vi "wd_replaceAll (STR).vi"(7 "data":string[](array[string]), 8 "error in (no error)":errorcluster, 9 "channel index":i32, 10 "data type":T7, 11 "meta in":T1={"TargetFile"=path "", "StreamMode"=enum."File", "Append?"=FALSE, "ChunkSize"=0, "TimeColumnMode"=enum."Empty", "TimestampFormat"="", "AbsoluteTime?"=FALSE, "FileAttribute "={"Creator"="", "Title"="", "SheetName"=""}, "Column"=[], "FileRef"=refnum, "MemoryRef"=[], "RecordInfo"=[], " ChannelPreviousInfo"=[], "ChannelFirstRecord"=[], "PredefinedFormattedValueLength"=20, "DiskTemplate"={"XMLRef"=[refnum, refnum, refnum, refnum, refnum, refnum], "ZipPath"=path "", "MetaFile"={"Ref"=refnum, "NextRow"=0, "NextPosition"=0, "Block"=[]}, "TempFolder"=path ""}}) -> (0 "error out":errorcluster, 3 "meta out":T1={"TargetFile"=path "", "StreamMode"=enum."File", "Append?"=FALSE, "ChunkSize"=0, "TimeColumnMode"=enum."Empty", "TimestampFormat"="", "AbsoluteTime?"=FALSE, "FileAttribute "={"Creator"="", "Title"="", "SheetName"=""}, "Column"=[], "FileRef"=refnum, "MemoryRef"=[], "RecordInfo"=[], " ChannelPreviousInfo"=[], "ChannelFirstRecord"=[], "PredefinedFormattedValueLength"=20, "DiskTemplate"={"XMLRef"=[refnum, refnum, refnum, refnum, refnum, refnum], "ZipPath"=path "", "MetaFile"={"Ref"=refnum, "NextRow"=0, "NextPosition"=0, "Block"=[]}, "TempFolder"=path ""}})   [LabVIEW 2017, in "NI_ExcelFile.lvlib"]
uses:
  <vilib>/express/express shared/NI_ExcelFile/NI_ExcelFile.lvlib
  <vilib>/express/express shared/NI_ExcelFile/Ctrls/DataType.ctl
  <vilib>/express/express shared/NI_ExcelFile/Ctrls/MainData.ctl
  <vilib>/express/express shared/NI_ExcelFile/Ctrls/StreamMode.ctl
  <vilib>/express/express shared/NI_ExcelFile/Ctrls/TimeColumnMode.ctl
  <vilib>/express/express shared/NI_ExcelFile/Ctrls/FileAttribute.ctl
  <vilib>/express/express shared/NI_ExcelFile/Ctrls/Columns.ctl
  <vilib>/express/express shared/NI_ExcelFile/Ctrls/ColumnInfo.ctl
  <vilib>/express/express shared/NI_ExcelFile/Ctrls/wd_recordInfo.ctl
  <vilib>/express/express shared/NI_ExcelFile/Ctrls/disk_TemplateFile.ctl
  <vilib>/express/express shared/NI_ExcelFile/Ctrls/meta_file.ctl
  <vilib>/express/express shared/NI_ExcelFile/Ctrls/meta_Block.ctl
  <vilib>/express/express shared/NI_ExcelFile/Ctrls/meta_BlockType.ctl
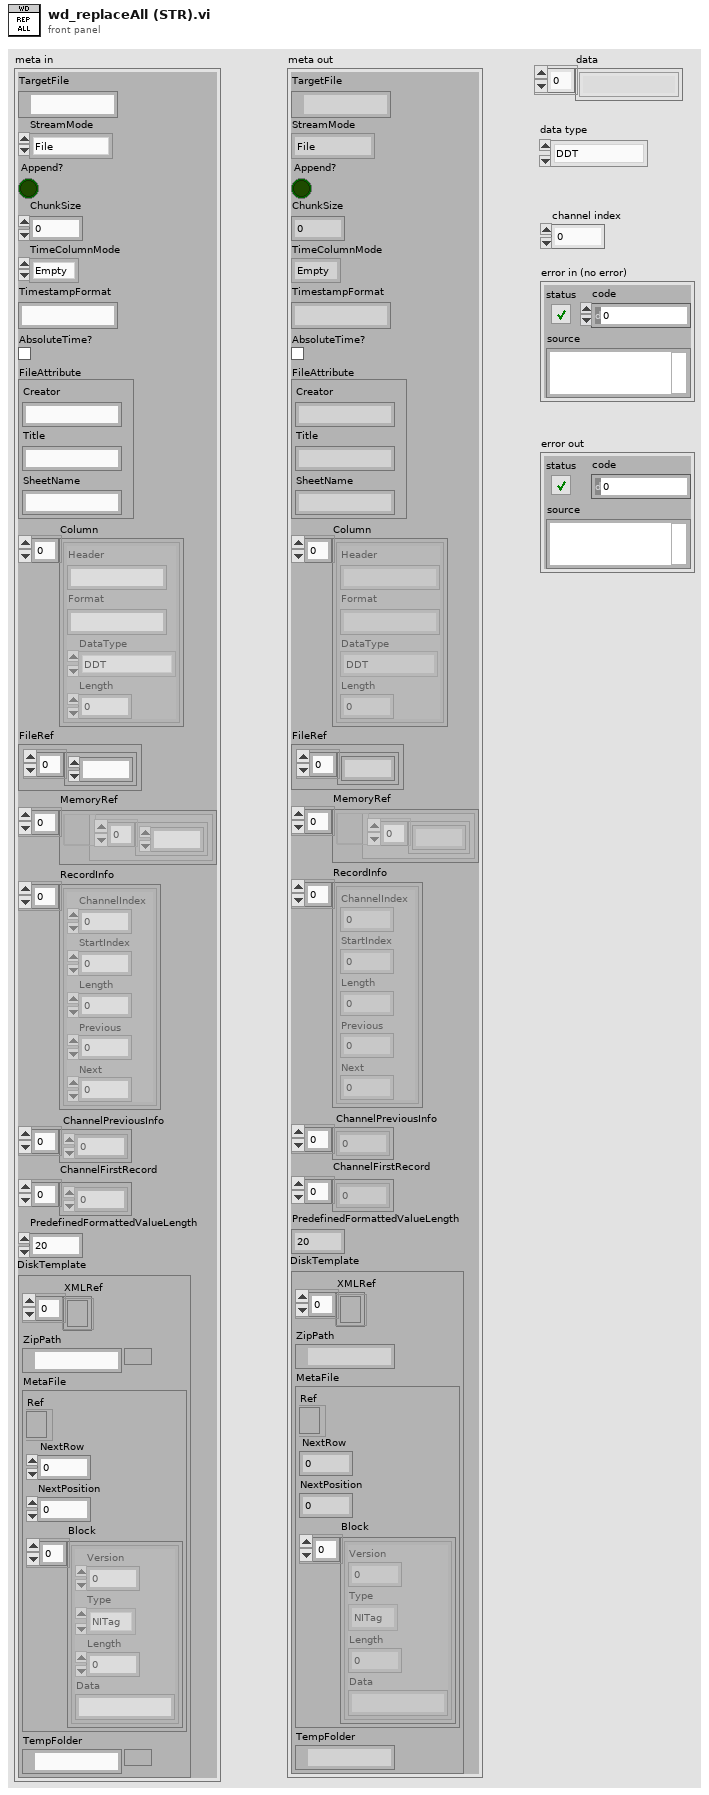
[diagram p1: front panel]
types:
  T1 = typedef "NI_ExcelFile.lvlib/MainData.ctl" = cluster{"TargetFile":path, "StreamMode":T2, "Append?":bool, "ChunkSize":u64, "TimeColumnMode":T3, "TimestampFormat":string, "AbsoluteTime?":bool, "FileAttribute ":T4, "Column":T5, "FileRef":refnum<k1>, "MemoryRef":refnum<data-value>[], "RecordInfo":T8[], " ChannelPreviousInfo":u32[], "ChannelFirstRecord":u32[], "PredefinedFormattedValueLength":i64, "DiskTemplate":T9}
  T2 = typedef "NI_ExcelFile.lvlib/StreamMode.ctl" = enum16{"File", "Memory"}
  T3 = typedef "NI_ExcelFile.lvlib/TimeColumnMode.ctl" = enum16{"Empty", "OnePerCh", "One"}
  T4 = typedef "NI_ExcelFile.lvlib/FileAttribute.ctl" = cluster{"Creator":string, "Title":string, "SheetName":string}
  T5 = typedef "NI_ExcelFile.lvlib/Columns.ctl" = T6[]
  T6 = typedef "NI_ExcelFile.lvlib/ColumnInfo.ctl" = cluster{"Header":string, "Format":string, "DataType":T7, "Length":u64}
  T7 = typedef "NI_ExcelFile.lvlib/DataType.ctl" = enum16{"DDT", "WFM", "Array of STR", "Array of DBL", "Array of I8", "Array of I16", "Array of I32", "Array of I64", "Array of SGL", "Array of U8", "Array of U16", "Array of U32", "Array of U64", "Array of Time"}
  T8 = typedef "NI_ExcelFile.lvlib/wd_recordInfo.ctl" = cluster{"ChannelIndex":u32, "StartIndex":u64, "Length":u64, "Previous":i32, "Next":i32}
  T9 = typedef "NI_ExcelFile.lvlib/disk_TemplateFile.ctl" = cluster{"XMLRef":refnum<file>[], "ZipPath":path, "MetaFile":T10, "TempFolder":path}
  T10 = typedef "NI_ExcelFile.lvlib/meta_file.ctl" = cluster{"Ref":refnum<file>, "NextRow":i32, "NextPosition":i64, "Block":T11[]}
  T11 = typedef "NI_ExcelFile.lvlib/meta_Block.ctl" = cluster{"Version":u16, "Type":T12, "Length":i32, "Data":string}
  T12 = typedef "NI_ExcelFile.lvlib/meta_BlockType.ctl" = enum16{"NITag", "File", "Column"}
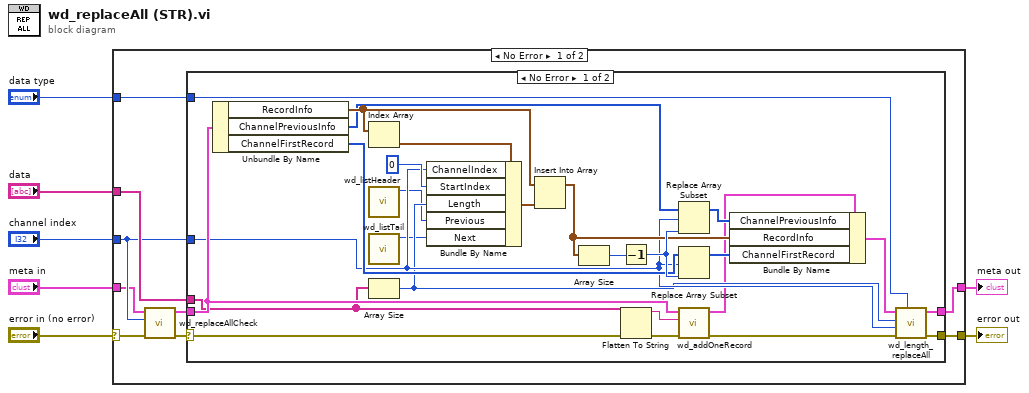
[diagram p0: block diagram]
diagram:
  n1 = case shown="No Error" "error in (no error)" {
    selector: "error in (no error)" -> [w8 w46]
    tunnel: "data type" -> [w13 _]
    tunnel: "channel index" -> [w12 _]
    tunnel: [w16 w45] -> w5
    tunnel: [w15 w46] -> w4
    tunnel: "data" -> [w14 _]
    tunnel: "meta in" -> [w11 w45]
    frame No Error {
      n2 = call <vilib>:"wd_replaceAllCheck.vi"("error in (no error)"=w8, "channel index"=w12, "meta in"=w11) -> ("error out"=w9:errorcluster, "meta out"=w10:T1)  [unwired: 7 in]
      n3 = case shown="No Error" w9 {
        selector: w9 -> [w21 w43]
        tunnel: [w22 w44] -> w16
        tunnel: [w19 w43] -> w15
        tunnel: w14 -> [w30 _]
        tunnel: w10 -> [w31 w44]
        tunnel: w13 -> [w25 _]
        tunnel: w12 -> [w27 _]
        frame No Error {
          n4 = Unbundle By Name(w31) -> ("RecordInfo"=w36:T8[], "ChannelPreviousInfo"=w33:u32[], "ChannelFirstRecord"=w32:u32[])
          n5 = Index Array(array=w36) -> (element=w34:T8)  [unwired: 1 in]
          n6 = call <vilib>:"wd_listHeader.vi"() -> ("list header"=w18:i32)  [unwired: 11 in]
          n7 = call <vilib>:"wd_listTail.vi"() -> ("list tail"=w17:i32)  [unwired: 11 in]
          n8 = Array Size(array=w30) -> (size(s)=w26:i32)
          n9 = Bundle By Name(cluster=w34, "ChannelIndex"=w27, "StartIndex"=u64 0 ("Start Index"), "Length"=w26, "Previous"=w18, "Next"=w17) -> (w37:T8)
          n10 = Insert Into Array(array=w36, new element=w37) -> (w40:T8[])  [unwired: 1 in]
          n11 = Array Size(array=w40) -> (size(s)=w38:i32)
          n12 = Decrement(x=w38) -> (x-1=w41:i32)
          n13 = Flatten To String(anything=w30, error in (no error)=w21) -> (data string=w29:string, error out=w28:errorcluster)  [unwired: 2 in, 1 out]
          n14 = Replace Array Subset(array=w33, new element=w41, index=w27) -> (w39:u32[])
          n15 = Replace Array Subset(array=w32, new element=w41, index=w27) -> (w42:u32[])
          n16 = call <vilib>:"wd_addOneRecord.vi"("error in (no error)"=w28, "data"=w29, "meta in"=w31) -> ("error out"=w20:errorcluster, "meta out"=w24:T1)  [unwired: 7 in]
          n17 = Bundle By Name(cluster=w24, "ChannelPreviousInfo"=w39, "RecordInfo"=w40, "ChannelFirstRecord"=w42) -> (w23:T1)
          n18 = call <vilib>:"wd_length_replaceAll.vi"("data type"=w25, "error in (no error)"=w20, "channel index"=w27, "size"=w26, "meta in"=w23) -> ("error out"=w19:errorcluster, "meta out"=w22:T1)  [unwired: 5 in]
        }
        frame Error {
        }
      }
    }
    frame Error {
    }
  }
  "error out" <- w4
  "meta out" <- w5
